vi "_UnitTest.enumpatch.vi"() -> ()   [LabVIEW 2017]
panel:
  in  "Cluster 3":T1={"enum"="a", "enum 2"="c", "str"="", "numeric"=0}
  in  "Cluster 2":T2={"enum"=2, "enum 2"=0, "str"="", "numeric"=0}
  in  "Cluster":T3={"enum"=enum."b", "enum 2"=enum."c", "str"="", "numeric"=0}
  out "data 3":T3={"enum"=enum."c", "enum 2"=enum."b", "str"="", "numeric"=0}
  out "data 2":T3={"enum"=enum."c", "enum 2"=enum."b", "str"="", "numeric"=0}
  out "data":T3={"enum"=enum."c", "enum 2"=enum."b", "str"="", "numeric"=0}
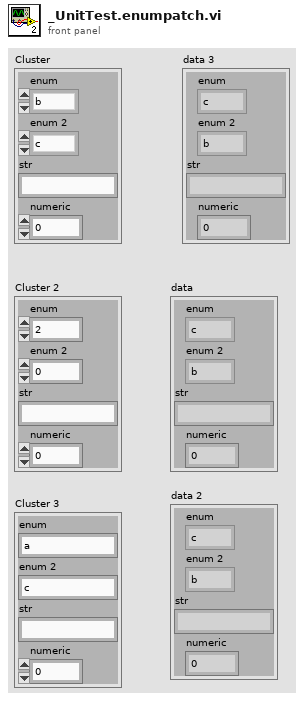
[diagram p1: front panel]
types:
  T1 = cluster{"enum":string, "enum 2":string, "str":string, "numeric":i32}
  T2 = cluster{"enum":i32, "enum 2":i32, "str":string, "numeric":i32}
  T3 = cluster{"enum":enum16{"a", "b", "c", "d"}, "enum 2":enum16{"a", "b", "c", "d"}, "str":string, "numeric":i32}
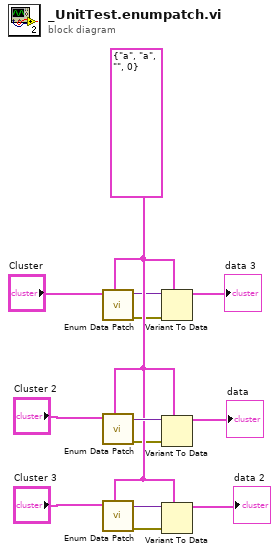
[diagram p0: block diagram]
diagram:
  w6 = T3 {"enum"=enum."a", "enum 2"=enum."a", "str"="", "numeric"=0}
  n1 = call "Enum Data Patch.vi"("Ref"=w6, "data in"="Cluster") -> ("error out"=w5:errorcluster, "data out"=w4:variant)  [unwired: 8 in]
  n2 = call "Enum Data Patch.vi"("Ref"=w6, "data in"="Cluster 2") -> ("error out"=w2:errorcluster, "data out"=w12:variant)  [unwired: 8 in]
  n3 = call "Enum Data Patch.vi"("Ref"=w6, "data in"="Cluster 3") -> ("error out"=w1:errorcluster, "data out"=w10:variant)  [unwired: 8 in]
  n4 = Variant To Data(error in=w5, type=w6, Variant=w4) -> (data=→"data 3":T3)  [unwired: 1 out]
  n5 = Variant To Data(error in=w2, type=w6, Variant=w12) -> (data=→"data":T3)  [unwired: 1 out]
  n6 = Variant To Data(error in=w1, type=w6, Variant=w10) -> (data=→"data 2":T3)  [unwired: 1 out]
